vi "read.vi"(7 "timeout (ms)":i32, 8 "error in (no error)":errorcluster, 9 "number of channels":i32, 10 "block size":i32, 11 "FPGAWrapperRK120511Fiber_Spiral in":refnum<class "FPGAWrapperRK110512Fiber_Spiral.lvclass">) -> (0 "error out":errorcluster, 1 "channels raw data block":T1, 2 "FIFO full?":bool, 3 "FPGAWrapperRK120511Fiber_Spiral out":refnum<class "FPGAWrapperRK110512Fiber_Spiral.lvclass">, 4 "timed out?":bool)   [LabVIEW 2010, in "FPGAWrapperRK110512Fiber_Spiral.lvclass"]
uses:
  FPGAWrapperRK110512Fiber_Spiral.lvclass
  common/arrays/pixel_raw_data_array.ctl
  GenericFPGAWrapper/GenericFPGAWrapper/GenericFPGAWrapper.lvclass
  <vilib>/rvi/interface/nirviReadWriteControl/nirviReadWriteControl.xnode
  FPGA_VI_Reference.ctl
  <vilib>/rvi/interface/common/niFpgaNodeNameForErrorReporting.ctl
  <vilib>/rvi/errors/niLvFpgaWhatHappensToTopLevelVI.ctl
  <vilib>/rvi/interface/nirviMethod/nirviMethod.xnode
  <vilib>/Utility/error.llb/Error Cluster From Error Code.vi
  <vilib>/rvi/errors/niLvFpgaAdjustHostInterfaceError.vi
  NiFpgaLv.dll
panel:
  out "elements remaining FIFO_2":u32
  out "elements remaining FIFO_1":u32
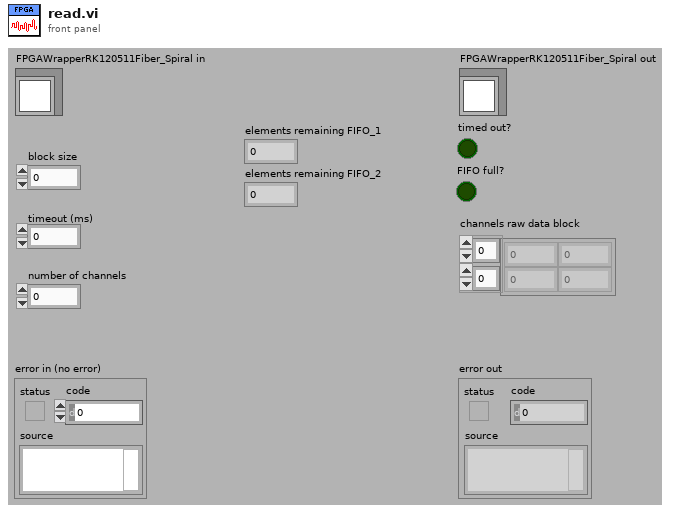
[diagram p1: front panel]
types:
  T1 = typedef "pixel_raw_data_array.ctl" = dbl[][]
  T2 = typedef "niFpgaNodeNameForErrorReporting.ctl" = enum16{"Open FPGA VI Reference", "Read/Write Control", "Invoke Method: Abort", "Invoke Method: Acknowledge IRQ", "Invoke Method: Download", "Invoke Method: FIFO.Configure", "Invoke Method: FIFO.Read", "Invoke Method: FIFO.Start", "Invoke Method: FIFO.Stop", "Invoke Method: FIFO.Write", "Invoke Method: Reset", "Invoke Method: Run", "Invoke Method: Wait on IRQ", "Close FPGA VI Reference"}
  T3 = typedef "niLvFpgaWhatHappensToTopLevelVI.ctl" = enum16{"top level VI scripted behind XNode", "top level VI inlined behind XNode"}
  T4 = typedef "FPGAWrapperRK110512Fiber_Spiral.lvclass/FPGA_VI_Reference.ctl" = refnum<k20>
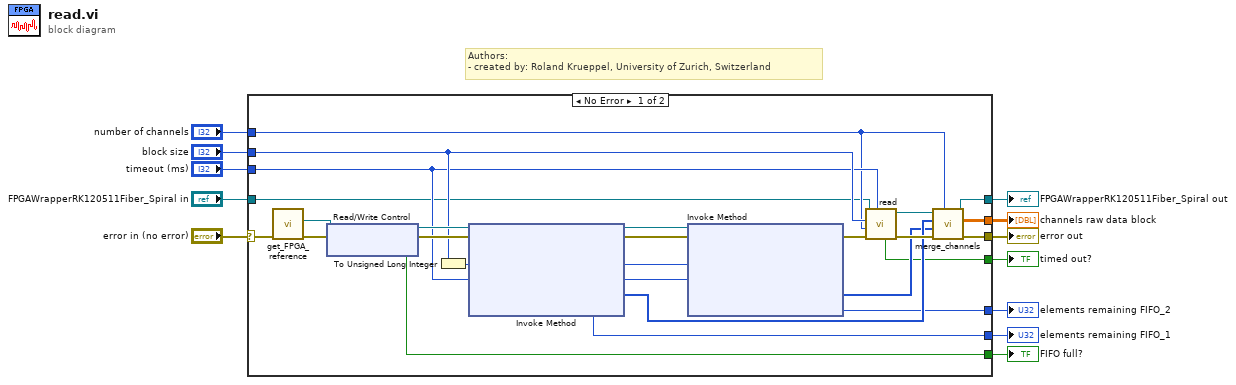
[diagram p0: block diagram]
diagram:
  # "Authors: \n- created by: Roland Krueppel, University of Zurich, Switzerland"
  n1 = case shown="No Error" "error in (no error)" {
    selector: "error in (no error)" -> [w36 w227]
    tunnel: "FPGAWrapperRK120511Fiber_Spiral in" -> [w13 w226]
    tunnel: [w33 _] -> w10
    tunnel: "timeout (ms)" -> [w25 _]
    tunnel: "block size" -> [w26 _]
    tunnel: "number of channels" -> [w18 _]
    tunnel: [w20 w227] -> w6
    tunnel: [w19 w226] -> w5
    tunnel: [w17 _] -> w4
    tunnel: [w16 _] -> w3
    tunnel: [w15 _] -> w2
    tunnel: [w14 _] -> w1
    frame No Error {
      n2 = call "get_FPGA_reference.vi"("error in (no error)"=w36) -> ("error out"=w34:errorcluster, "FPGA VI Reference"=w35:T4)  [unwired: 8 in, 1 out]
      n3 = xnode "Read/Write Control"("FPGA VI Reference In"=w35, "error in"=w34) -> ("FPGA VI Reference Out"=w31:T4, "error out"=w32:errorcluster, "FIFO overflow"=w33:bool)
      n4 = To Unsigned Long Integer(number=w26) -> (unsigned 32bit integer=w27:u32)
      n5 = xnode "Invoke Method"("FPGA VI Reference In"=w31, "error in"=w32, "Number of Elements"=w27, "Timeout (ms)"=w25) -> ("FPGA VI Reference Out"=w30:T4, "error out"=w29:errorcluster, "Data"=w22:u32[], "Elements Remaining"=w14:u32)
      n6 = xnode "Invoke Method"("FPGA VI Reference In"=w30, "error in"=w29, "Number of Elements"=w27, "Timeout (ms)"=w25) -> ("error out"=w28:errorcluster, "Data"=w21:u32[], "Elements Remaining"=w15:u32)  [unwired: 1 out]
      n7 = call-parent "read.vi"("timeout (ms)"=w25, "error in (no error)"=w28, "number of channels"=w18, "block size"=w26, "GenericFPGAWrapper in"=w13) -> ("error out"=w24:errorcluster, "FIFO full?"=w16:bool, "GenericFPGAWrapper out"=w23:refnum<class "FPGAWrapperRK110512Fiber_Spiral.lvclass">)  [unwired: 2 in, 2 out]
      n8 = call-dynamic "merge_channels.vi"("number of channels"=w18, "error in (no error)"=w24, "FIFO_2"=w21, "FIFO_1"=w22, "FPGAWrapperRK120511Fiber_Spiral in"=w23) -> ("error out"=w20:errorcluster, "channels raw data block"=w17:T1, "FPGAWrapperRK120511Fiber_Spiral out"=w19:refnum<class "FPGAWrapperRK110512Fiber_Spiral.lvclass">)  [unwired: 4 in]
    }
    frame Error {
    }
  }
  "error out" <- w6
  "FPGAWrapperRK120511Fiber_Spiral out" <- w5
  "FIFO full?" <- w10
  "channels raw data block" <- w4
  "timed out?" <- w3
  "elements remaining FIFO_1" <- w1
  "elements remaining FIFO_2" <- w2
